vi "ExpandComic.vi"(6 "Status":refnum<vi>, 8 "error in (no error)":errorcluster, 10 "Working Dir":path, 11 "Source":path) -> (0 "error out":errorcluster, 3 "Working Dir Out":path)   [LabVIEW 2022 SP3]
panel:
  out "resulting string":string
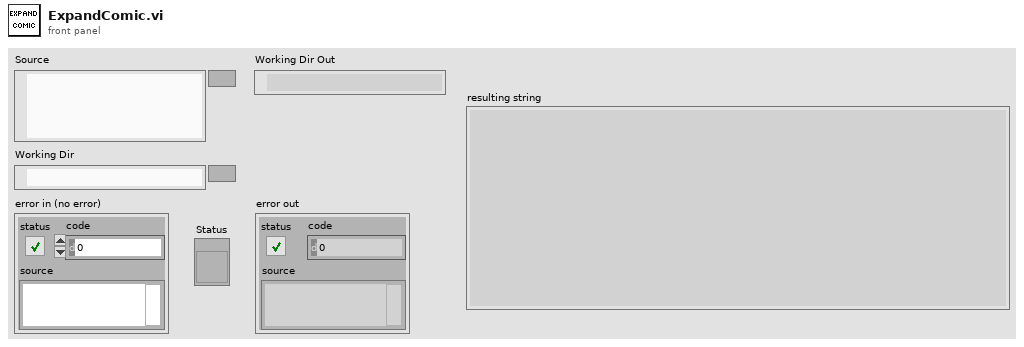
[diagram p1: front panel]
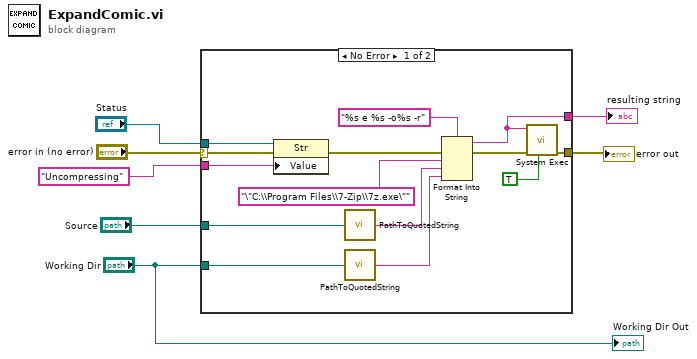
[diagram p0: block diagram]
diagram:
  n1 = case shown="No Error" "error in (no error)" {
    selector: "error in (no error)" -> [w8 w22]
    tunnel: [w21 w22] -> w7
    tunnel: [w18 _] -> w6
    tunnel: "Source" -> [w15 _]
    tunnel: "Working Dir" -> [w12 _]
    tunnel: "Status" -> [w10 _]
    tunnel: "Uncompressing" ("Value") -> [w9 _]
    frame No Error {
      n2 = property class="Str"(reference=w10, error in=w8, "Value"=w9) -> (error out=w11:errorcluster)  [unwired: 1 out]
      n3 = call "PathToQuotedString.vi"("Path"=w15) -> ("String"=w14:string)  [unwired: 4 in]
      n4 = call "PathToQuotedString.vi"("Path"=w12) -> ("String"=w16:string)  [unwired: 4 in]
      n5 = Format Into String(format string="%s e %s -o%s -r", error in=w11, "\"C:\\Program Files\\7-Zip\\7z.exe\"" ("input 1"), w14, w16) -> (resulting string=w18:string, error out=w19:errorcluster)  [unwired: 1 in]
      n6 = call <vilib>:"System Exec.vi"("run minimized? (F)"=TRUE, "error in (no error)"=w19, "command line"=w18) -> ("error out"=w21:errorcluster)  [unwired: 5 in, 3 out]
    }
    frame Error {
    }
  }
  "error out" <- w7
  "resulting string" <- w6
  "Working Dir Out" <- "Working Dir"
